vi "cblas dcopy.vi"(5 "n":i32=-1, 6 "incy":i32=1, 7 "incx":i32=1, 10 "y":dbl[](array[numeric]), 11 "x":dbl[](array[numeric])) -> (0 "error":i32, 3 "dcopy":dbl[](array[numeric]))   [LabVIEW 2018, in "NI_AALBLAS.lvlib"]
uses:
  NI_AALBLAS.lvlib
  <resource>/lvblas.dll
panel:
  # "void cblas_dcopy(n, *x, incx, *y, incy)"
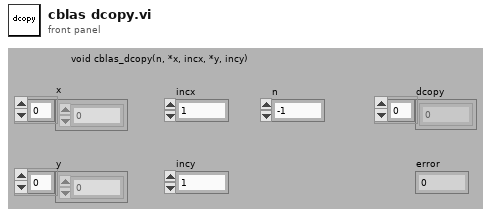
[diagram p1: front panel]
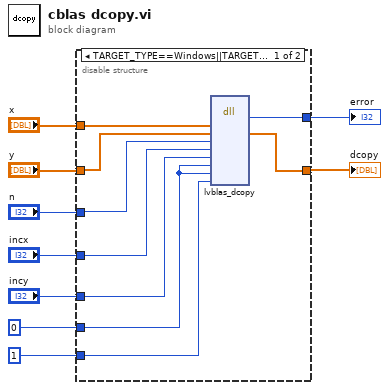
[diagram p0: block diagram]
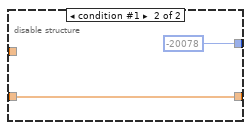
[diagram p2: hidden frame]
diagram:
  n1 = disable-structure shown="TARGET_TYPE==Windows||TARGET_TYPE==Unix||TARGET_TYPE==Mac||TARGET_TYPE==RT" {
    disable-tunnel: "y" -> [w17 w20]
    disable-tunnel: [w15 w20] -> w8
    disable-tunnel: [w16 -20078] -> w7
    disable-tunnel: "x" -> [w18 _]
    disable-tunnel: "n" -> [w14 _]
    disable-tunnel: "incx" -> [w13 _]
    disable-tunnel: "incy" -> [w12 _]
    disable-tunnel: 0 -> [w11 _]
    disable-tunnel: 1 -> [w10 _]
    frame condition #0 (active) {
      n2 = dll-call lib="C:/Program Files (x86)/National Instruments/LabVIEW 2018/resource/lvblas.*" fn="lvblas_dcopy" ("LVBLAS.dll:BLASCopyVectorH")("X"=w18, "Y"=w17, "N"=w14, "IncX"=w13, "IncY"=w12, "startX"=w11, "startY"=w11, "check"=w10) -> ("error"=w16:i32, "Y"=w15:dbl[])  [unwired: 10 in, 2 out]
    }
    frame condition #1 {
    }
  }
  "dcopy" <- w8
  "error" <- w7
